vi "Fetch Data from 5772 (Raw Data)_4xI16.vi"(7 "Timeout (s)":i32=5, 8 "error in":errorcluster, 10 "Samples":i32=-1, 11 "FPGA VI Reference In":refnum<k20>) -> (0 "error out":errorcluster, 2 "Data Acquired":i16[](array[numeric]), 3 "FPGA VI Reference Out":refnum<k20>, 4 "Elements Remaining":u32)   [LabVIEW 2012]
uses:
  <vilib>/Utility/error.llb/Error Cluster From Error Code.vi
  <vilib>/rvi/errors/niLvFpgaAdjustHostInterfaceError.vi
  <vilib>/rvi/interface/nirviMethod/nirviMethod.xnode
  <vilib>/FPGAPlugInAG/Dynamic/niLvFpga_ReadFifo_Dynamic.vi
  <vilib>/rvi/errors/niLvFpgaMergeErrorWithErrorCode.vi
panel:
  in  "FIFO Type":enum16{"FPGA to Host FIFO (U64)", "Generic"}(ring)
  out "Data":i16[](array[numeric])
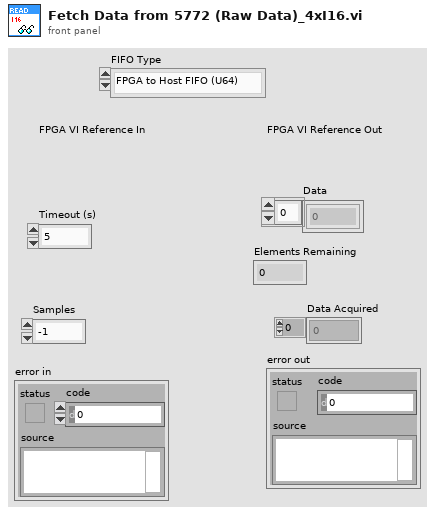
[diagram p1: front panel]
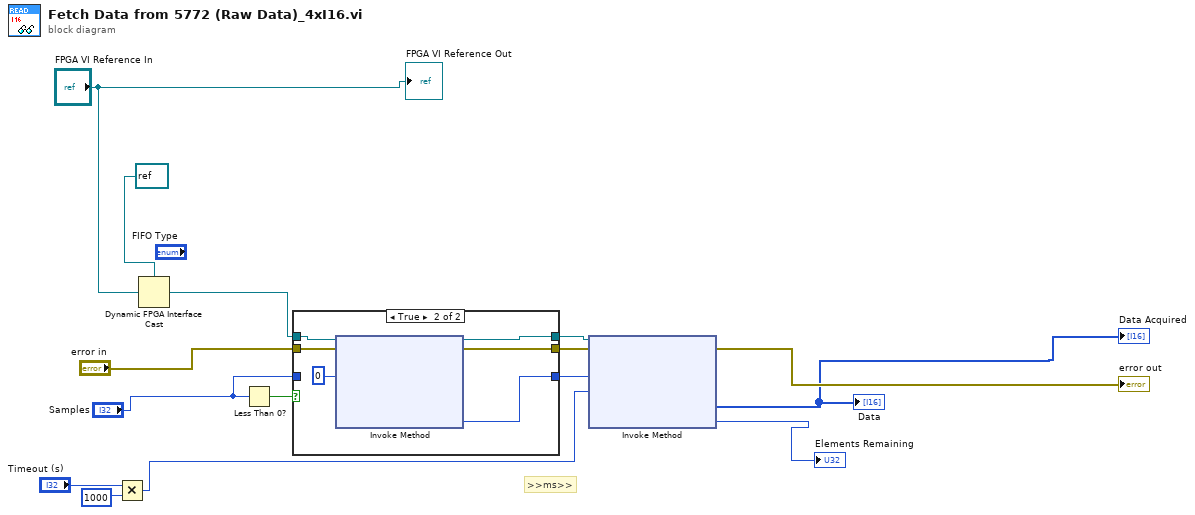
[diagram p0: block diagram]
diagram:
  # ">>ms>>"
  n1 = Multiply(x="Timeout (s)", y=1000) -> (x*y=w10:i32)
  n2 = Dynamic FPGA Interface Cast(Session In=refnum<k20> refnum ("Type"), Type="FPGA VI Reference In") -> (Session Out=w14:refnum<k20>)
  n3 = Less Than 0?(x="Samples") -> (x < 0?=w4:bool)
  n4 = case shown="True" w4 {
    tunnel: w14 -> [w18 w24]
    tunnel: "error in" -> [w17 w23]
    tunnel: [w18 w22] -> w3
    tunnel: [w17 w21] -> w2
    tunnel: [w16 w20] -> w1
    tunnel: "Samples" -> [w16 _]
    frame False {
    }
    frame True {
      n5 = xnode "Invoke Method"("FPGA VI Reference In"=w24, "error in"=w23, "Number of Elements"=u32 0) -> ("FPGA VI Reference Out"=w22:refnum<k20>, "error out"=w21:errorcluster, "Elements Remaining"=w20:u32)  [unwired: 1 in, 1 out]
    }
  }
  n6 = xnode "Invoke Method"("FPGA VI Reference In"=w3, "error in"=w2, "Number of Elements"=w1, "Timeout (ms)"=w10) -> ("error out"=→"error out":errorcluster, "Data"=→"Data Acquired" →"Data":i16[], "Elements Remaining"=→"Elements Remaining":u32)  [unwired: 1 out]
  "FPGA VI Reference Out" <- "FPGA VI Reference In"
